vi "未命名 3.vi"() -> ()   [LabVIEW 2012]
panel:
  in  "数值":i32
  in  "文件（使用对话框）":path
  in  "停止":bool
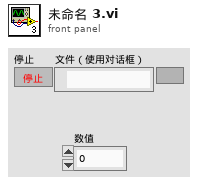
[diagram p1: front panel]
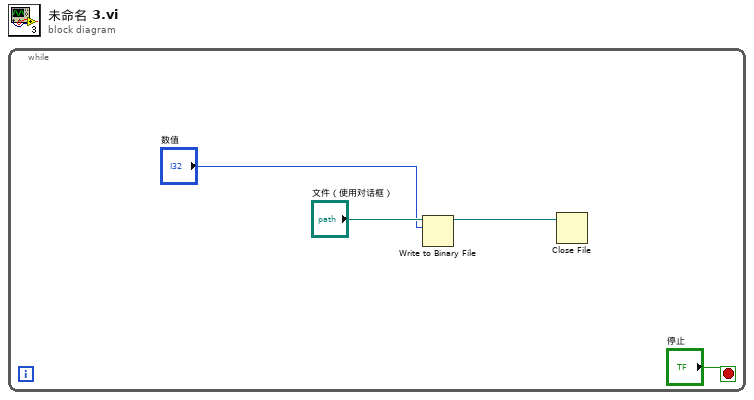
[diagram p0: block diagram]
diagram:
  n1 = while {
    stop <- "停止" stop-if-true
    n2 = Write to Binary File(file (use dialog)="文件（使用对话框）", data="数值") -> (refnum out=w2:refnum<file>)  [unwired: 4 in, 2 out]
    n3 = Close File(refnum=w2) -> ()  [unwired: 1 in, 2 out]
  }
